vi "niScope Multi Record.vi"() -> ()   [LabVIEW 2020]
doc: "Example: Multi Record\n\nRecommended Input Signal: 100 kHz, 8 Vpp, sine wave\n\nDevices Supported: Refer to NI Example Finders\n\nLabVIEW Description:\n\nThis VI demonstrates the multi-record capabilities of National Instruments high-speed oscilloscope. In a multi-record acquisition, each record is one waveform with at least \"min record length\" points as specified with the Configure Horizontal Timing VI. Furthermore, each record is triggered, so when the trigger arrives for the first record, the hardware quickly rearms for the next record. All records are stored in the onboard memory until they are retrieved with the Fetch VI. In this example, the Fetch VI has a positive timeout value, which pauses the program until all records have been acquired into the onboard memory before it fetches the waveforms.\n\nIf the \"plot relative to\" parameter is set to trigger, all records are overlaid on the same graph with the trigger occurring at time zero for each waveform. Notice that the points do not line up in time from different acquisitions. This is due to a very accurate measurement of the trigger time -- much more accurate than the time between two samples. The trigger time measurement is included in the relative initial x value, which is the time from the first sample to the trigger. It is returned by the Fetch VI. This accurate trigger time measurement is what allows random interleaved sampling to work. \n\nIf the \"plot relative to\" parameter is set to absolute, the records are all plotted on the same time scale. This feature is only available on oscilloscopes that support continuous acquisition. Using the absolute time scale, you will see the dead time, in which no points are acquired, between records. This allows you to compute the time between two records to the accuracy of the oscilloscope's sample clock. The absolute time is made possible by a free running, 48-bit counter on the oscilloscope. This counter is only cleared with the Reset, Abort, or Close VIs. Therefore, you could even use the absolute timestamp to compare the time between two software initiated acquisitions - the dead time would just be much longer. Refer to the NI High Speed Digitizers Help for more information about timestamps."
uses:
  <instrlib>/niScope/Controls/niScope trigger source digital.ctl
  <instrlib>/niScope/Controls/niScope vertical coupling.ctl
  <vilib>/Analysis/baseanly.llb/Mean (DBL).vi
  <instrlib>/niScope/Configure/Trigger/niScope Configure Trigger Digital.vi
  <instrlib>/niScope/Acquire/Fetch/niScope Multi Fetch.vi
  <vilib>/Analysis/NI_AALBase.lvlib
panel:
  in  "Color Picker":u32(colorbox)
  in  "Plot Color Mode":u16(ring) items=["Random", "Selected Color"]
  in  "Plot Relative To":u16(ring)=1 items=["Absolute", "Trigger"]
  in  "Plot Style":u16(ring) items=["Lines", "Points"]
  in  "Number Of Records":i32=3
  out "Waveform Graph":T1(graph)=[{"relativeInitialX"=-4e-06, "xIncrement"=8e-10, "wfm"=array[10000 elements]}, {"relativeInitialX"=-4e-06, "xIncrement"=8e-10, "wfm"=array[10000 elements]}, {"relativeInitialX"=-4e-06, "xIncrement"=8e-10, "wfm"=array[10000 elements]}, {"relativeInitialX"=-4e-06, "xIncrement"=8e-10, "wfm"=array[10000 elements]}]
  in  "Min. Record Length":i32=10000
  in  "Min. Sample Rate":dbl=1250000000.0 step=1000000.0 format="%#.3p"
  in  "Vertical Range (V)":dbl=0.1 format="%#.2p"
  in  "Channel Name":string="0,1"
  in  "Resource Name":refnum<k15>="scope" caption="Resource Name(s)"
  # "Overview: Demonstrates some of the advanced measurement library functions such as waveform processing.\nRequirements: NI-SCOPE\nInstructions: \n1.  Select the appropriate device in the Resource Name control.\n2.  Enter the channel you would like to acquire from in the Channel Name control.\n3.  Run the VI."
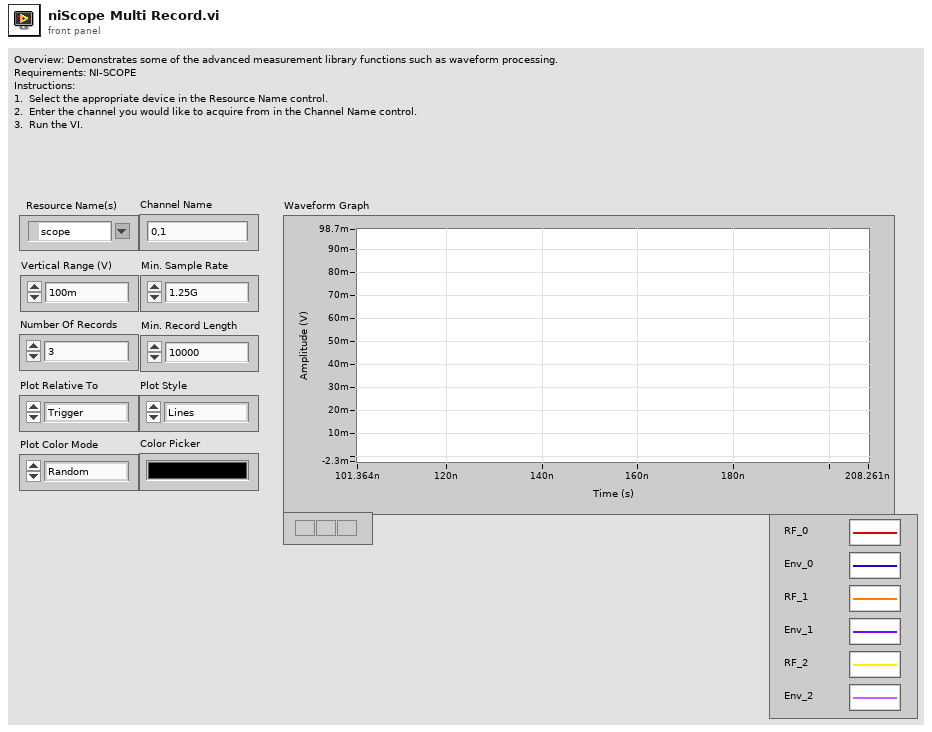
[diagram p1: front panel]
types:
  T1 = cluster{"relativeInitialX":dbl, "xIncrement":dbl, "wfm":dbl[]}[]
  T2 = typedef "niScope vertical coupling.ctl" = i32
  T3 = typedef "niScope trigger source digital.ctl" = string
  T4 = cluster{"actualSamples":i32, "absoluteInitialX":dbl, "relativeInitialX":dbl, "xIncrement":dbl, "offset":dbl, "gain":dbl, "reserved1":dbl, "reserved2":dbl}[]
  T5 = cluster{"absoluteInitialX":dbl, "xIncrement":dbl, "wfm":dbl[]}
  T6 = cluster{"relativeInitialX":dbl, "xIncrement":dbl, "wfm":dbl[]}
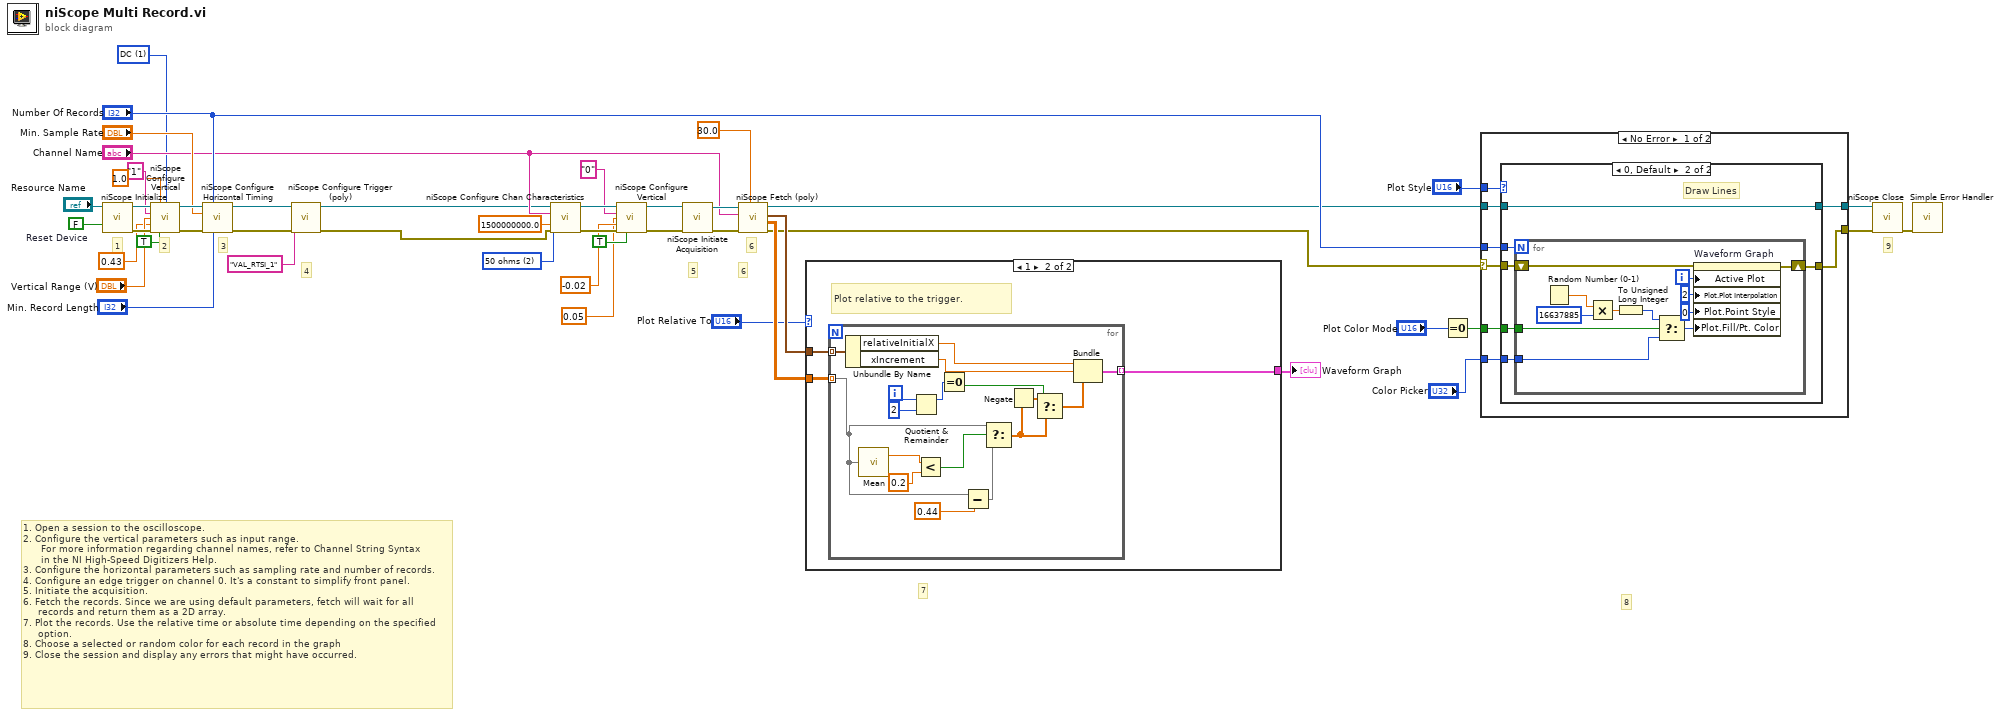
[diagram p0: block diagram]
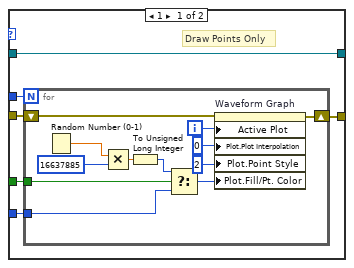
[diagram p2: hidden frame]
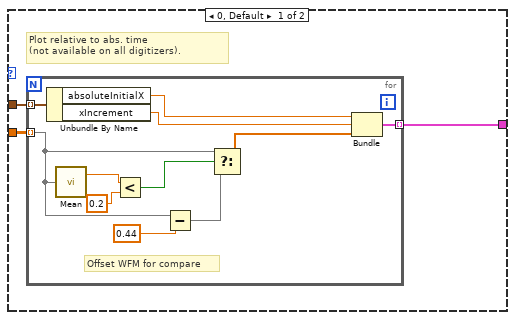
[diagram p4: hidden frame]
diagram:
  w1 = T2 1 items=["AC", "DC", "Ground"] ("vertical coupling")
  w17 = u32 2 items=["1 mega ohm"=0, "50 ohms"=2] ("input impedance")
  w47 = FALSE  # Reset Device
  # "6"
  # "1. Open a session to the oscilloscope.\n2. Configure the vertical parameters such as input range.\n      For more information regarding channel names, refer to Channel String Syntax \n      in the NI High-Speed Digitizers Help.\n3. Configure the horizontal parameters such as sampling rate and number of records.\n4. Configure an edge trigger on channel 0. It's a constant to simplify front panel.\n5. Initiate the acquisition.\n6. Fetch the records. Since we are using default parameters, fetch will wait for all\n     records and return them as a 2D array.\n7. Plot the records. Use the relative time or absolute time depending on the specified\n     option.\n8. Choose a selected or random color for each record in the graph\n9. Close the session and display any errors that might have occurred."
  # "9"
  # "8"
  # "7"
  # "6"
  # "5"
  # "4"
  # "3"
  # "2"
  # "1"
  n1 = call <instrlib>:"niScope Initialize.vi"("resource name"="Resource Name", "reset device"=w47) -> ("instrument handle"=w41:refnum<k15>, "error out"=w40:errorcluster)  [unwired: 12 in]
  n2 = call <instrlib>:"niScope Configure Vertical.vi"("instrument handle"=w41, "probe attenuation"=1.0, "vertical coupling"=w1, "channels"="1", "vertical range"="Vertical Range (V)", "vertical offset"=0.43, "error in"=w40, "channel enabled"=TRUE) -> ("instrument handle out"=w44:refnum<k15>, "error out"=w45:errorcluster)  [unwired: 6 in]
  n3 = call <instrlib>:"niScope Configure Horizontal Timing.vi"("instrument handle"=w44, "number of records"="Number Of Records", "min sample rate"="Min. Sample Rate", "error in"=w45, "min record length"="Min. Record Length") -> ("instrument handle out"=w37:refnum<k15>, "error out"=w38:errorcluster)  [unwired: 9 in]
  n4 = call-poly <instrlib>:"niScope Configure Trigger (poly).vi"("instrument handle"=w37, "trigger source"=T3 "VAL_RTSI_1", "error in"=w38) -> ("instrument handle out"=w2:refnum<k15>, "error out"=w33:errorcluster)  [unwired: 11 in]
  n5 = call <instrlib>:"niScope Configure Chan Characteristics.vi"("instrument handle"=w2, "channels"="Channel Name", "input impedance"=w17, "maximum input frequency"=1500000000.0, "error in"=w33) -> ("instrument handle out"=w14:refnum<k15>, "error out"=w18:errorcluster)  [unwired: 9 in]
  n6 = call <instrlib>:"niScope Configure Vertical.vi"("instrument handle"=w14, "channels"="0", "vertical range"=0.05, "vertical offset"=-0.02, "error in"=w18, "channel enabled"=TRUE) -> ("instrument handle out"=w13:refnum<k15>, "error out"=w15:errorcluster)  [unwired: 8 in]
  n7 = call <instrlib>:"niScope Initiate Acquisition.vi"("instrument handle"=w13, "error in"=w15) -> ("instrument handle out"=w31:refnum<k15>, "error out"=w32:errorcluster)  [unwired: 12 in]
  n8 = call-poly <instrlib>:"niScope Fetch (poly).vi"("timeout"=30.0, "error in"=w32, "channels"="Channel Name", "instrument handle"=w31) -> ("error out"=w25:errorcluster, "wfm"=w36:dbl[][], "wfm info"=w35:T4, "instrument handle out"=w30:refnum<k15>)  [unwired: 4 in]
  n9 = case shown="1" "Plot Relative To" {
    tunnel: w35 -> [w48 w62]
    tunnel: w36 -> [w50 w64]
    tunnel: [w49 w63] -> w34
    frame 0, Default {
      # "Plot relative to abs. time\n(not available on all digitizers)."
      n10 = for {
        tunnel: w50 -> [w53] mode=indexing
        tunnel: [w59] -> w49 mode=indexing
        tunnel: w48 -> [w58] mode=indexing
        # "Offset WFM for compare"
        n11 = Unbundle By Name(w58) -> ("absoluteInitialX"=w61:dbl, "xIncrement"=w60:dbl)
        n12 = call-poly <vilib>:"Mean.vi"("X"=w53) -> ("mean"=w57:dbl)  [unwired: 1 out]
        n13 = Less?(x=w57, y=0.2) -> (x < y?=w55:bool)
        n14 = Subtract(x=w53, y=0.44) -> (x-y=w51:dbl[])
        n15 = Select(t=w53, s=w55, f=w51) -> (s? t:f=w54:dbl[])
        n16 = Bundle("absoluteInitialX"=w61, "xIncrement"=w60, "wfm"=w54) -> (w59:T5)  [unwired: 1 in]
      }
    }
    frame 1 {
      # "Plot relative to the trigger."
      n17 = for {
        tunnel: w64 -> [w72] mode=indexing
        tunnel: [w79] -> w63 mode=indexing
        tunnel: w62 -> [w78] mode=indexing
        i -> [w71]
        n18 = Unbundle By Name(w78) -> ("relativeInitialX"=w81:dbl, "xIncrement"=w80:dbl)
        n19 = call-poly <vilib>:"Mean.vi"("X"=w72) -> ("mean"=w77:dbl)  [unwired: 1 out]
        n20 = Quotient & Remainder(x=w71, y=2) -> (x-y*floor(x/y)=w69:i32)  [unwired: 1 out]
        n21 = Less?(x=w77, y=0.2) -> (x < y?=w75:bool)
        n22 = Equal To 0?(x=w69) -> (x = 0?=w68:bool)
        n23 = Subtract(x=w72, y=0.44) -> (x-y=w73:dbl[])
        n24 = Select(t=w72, s=w75, f=w73) -> (s? t:f=w67:dbl[])
        n25 = Negate(x=w67) -> (-x=w66:dbl[])
        n26 = Select(t=w66, s=w68, f=w67) -> (s? t:f=w65:dbl[])
        n27 = Bundle("relativeInitialX"=w81, "xIncrement"=w80, "wfm"=w65) -> (w79:T6)  [unwired: 1 in]
      }
    }
  }
  "Waveform Graph" <- w34
  n28 = Equal To 0?(x="Plot Color Mode") -> (x = 0?=w22:bool)
  n29 = case shown="No Error" w25 {
    selector: w25 -> [w83 w126]
    tunnel: "Number Of Records" -> [w89 _]
    tunnel: w30 -> [w88 w127]
    tunnel: [w87 w127] -> w29
    tunnel: [w82 w126] -> w28
    tunnel: "Plot Style" -> [w86 _]
    tunnel: w22 -> [w85 _]
    tunnel: "Color Picker" -> [w84 _]
    frame No Error {
      n30 = case shown="0, Default" w86 {
        tunnel: w89 -> [w95 w113]
        tunnel: w88 -> [w94 w112]
        tunnel: [w94 w112] -> w87
        tunnel: w85 -> [w93 w111]
        tunnel: w84 -> [w92 w110]
        tunnel: w83 -> [w91 w109]
        tunnel: [w90 w108] -> w82
        frame 1 {
          # "Draw Points Only"
          n31 = for {
            N: w95 -> [_]
            tunnel: w93 -> [w103]
            tunnel: w92 -> [w99]
            shift-right: [w96] -> w90
            shift-left: w91 -> [w97]
            i -> [w107]
            n32 = Random Number (0-1)() -> (number: 0 to 1=w101:dbl)
            n33 = Multiply(x=w101, y=u32 16637885 ("Y")) -> (x*y=w100:dbl)
            n34 = To Unsigned Long Integer(number=w100) -> (unsigned 32bit integer=w98:u32)
            n35 = Select(t=w98, s=w103, f=w99) -> (s? t:f=w104:u32)
            n36 = property on="Waveform Graph" class="WFGraph (strict)"(error in=w97, "Active Plot"=w107, "Plot.Plot Interpolation"=u8 0 ("Write Attribute"), "Plot.Point Style"=u8 2 ("Write Attribute"), "Plot.Fill/Pt. Color"=w104) -> (error out=w96:errorcluster)  [unwired: 1 in, 1 out]
          }
        }
        frame 0, Default {
          # "Draw Lines"
          n37 = for {
            N: w113 -> [_]
            tunnel: w111 -> [w118]
            tunnel: w110 -> [w117]
            shift-right: [w114] -> w108
            shift-left: w109 -> [w115]
            i -> [w125]
            n38 = Random Number (0-1)() -> (number: 0 to 1=w121:dbl)
            n39 = Multiply(x=w121, y=u32 16637885 ("Y")) -> (x*y=w120:dbl)
            n40 = To Unsigned Long Integer(number=w120) -> (unsigned 32bit integer=w116:u32)
            n41 = Select(t=w116, s=w118, f=w117) -> (s? t:f=w119:u32)
            n42 = property on="Waveform Graph" class="WFGraph (strict)"(error in=w115, "Active Plot"=w125, "Plot.Plot Interpolation"=u8 2 ("Write Attribute"), "Plot.Point Style"=u8 0 ("Write Attribute"), "Plot.Fill/Pt. Color"=w119) -> (error out=w114:errorcluster)  [unwired: 1 in, 1 out]
          }
        }
      }
    }
    frame Error {
    }
  }
  n43 = call <instrlib>:"niScope Close.vi"("instrument handle"=w29, "error in"=w28) -> ("error out"=w27:errorcluster)  [unwired: 13 in]
  n44 = call <vilib>:"Simple Error Handler.vi"("error in (no error)"=w27) -> ()  [unwired: 4 in, 5 out]
